vi "ABFL2dll.vi"(8 "error in (no error)":errorcluster, 11 "ABFL2 Inputs":T2) -> (0 "error out":errorcluster, 3 "ABFL2 Outputs":T1)   [LabVIEW 2016]
doc: "subroutine ABFL2dll(a, b, z, kq, ksat, ab, tbub, tdew, pbub, pdew, dlbub, dvdew, ybub, xdew, t, p, dl, dv, x,\ny, q, ierr, herr, ab_length, herr_length)\n\nGeneral flash calculation given two inputs and composition. Valid properties for the first input are temperature,\npressure, and density. Valid properties for the second are pressure, density, energy, enthalpy, entropy, or quality.\nThe character string ab specifies the inputs.\n\nThis routine accepts only two-phase states as inputs; it is intended primarily for use by the general flash routines\nsuch as THFLSH or TSFLSH. It may be called independently if the state is known to be two-phase. But beware\n- this routine does not check limits, and it will be significantly faster than TSFLSH, etc., when the bubble and\ndew point limits can be provided (ksat=1 option).\n\nThis routine calls TPFL2 within a secant-method iteration to find a solution. Initial guesses are based on the\nliquid density at the bubble point and the vapor density at the dew point.\n\nINPUTS:\n\na -- First property (either temperature, pressure, or density)\nb -- Second property (pressure, density, energy, enthalpy, entropy, or quality)\nz -- Overall composition (array of mole fractions)\nkq -- Flag specifying units for input quality when b=quality:\nksat -- Flag for bubble and dew point limits:\nab -- Character*2 string defining the inputs, e.g., 'TD' or 'PQ'\ntbub -- Bubble point temperature [K] at (P and x=z)\ntdew -- Dew point temperature [K] at (P and y=z) For temperature inputs:\npbub -- Bubble point pressure [kPa] at (T and x=z)\npdew -- Dew point pressure [kPa] at (T and y=z) For either case:\nDlbub -- Liquid density [mol/L] at bubble point\nDvdew -- Vapor density [mol/L] at dew point\nybub -- Vapor composition (array of mole fractions) at bubble point\nxdew -- Liquid composition (array of mole fractions) at dew point\nt -- Temperature [K] (if not an input)\np -- Pressure [kPa] (if not an input) \n\nOUTPUTS:\n\nt -- Temperature [K] (if not an input)\np -- Pressure [kPa] (if not an input) \n\nAll other output variables (starting with Dl) are given in the ABFLASH routine.\n\nDl -- molar density [mol/L] of the liquid phase\nDv -- molar density [mol/L] of the vapor phase \nx -- composition of liquid phase [array of mol frac]\ny -- composition of vapor phase [array of mol frac] \nq -- vapor quality on a MOLAR basis [moles vapor/total moles]\n q < 0 indicates subcooled (compressed) liquid\n q = 0 indicates saturated liquid\n q = 1 indicates saturated vapor\n q > 1 indicates superheated vapor\n q = 998 superheated vapor, but quality not defined (in most situations, t > Tc)\n q = 999 indicates supercritical state (t > Tc) and (p > Pc)\nierr -- Error flag\nherr -- Error string (character*255 variable if ierr<>0)\nab_length -- length of variable ab (default: 2)\nherr_length -- length of variable herr (default: 255)\n\nFLAGS:\n \nkq flags\n 1 Quality on molar basis (moles vapor/total moles)\n 2 Quality on mass basis (mass vapor/total mass)\nksat flags\n 1 Must provide values for the following:\n 0 Dew and bubble point limits computed here\nierr flags\n 0 Successful\n 224 Dew point calculation did not converge\n 223 Bubble point calculation did not converge\n 226 2-phase iteration did not converge"
uses:
  REFPROP.DLL
panel:
  # "REFPROP-ABFL2dll.vi"
  # "void  ABFL2dll(double *a, double *b, double *z, int32_t *kq, int32_t *ksat, CStr ab, double *tbub, double *tdew, double *pbub, double *pdew, double *Dlbub, double *Dvdew, double *ybub, double *xdew, double *t, double *p, double *Dl, double *Dv, double *x, double *y, double *q, int32_t *ierr, CStr herr, int32_t ab_length, int32_t herr_length)"
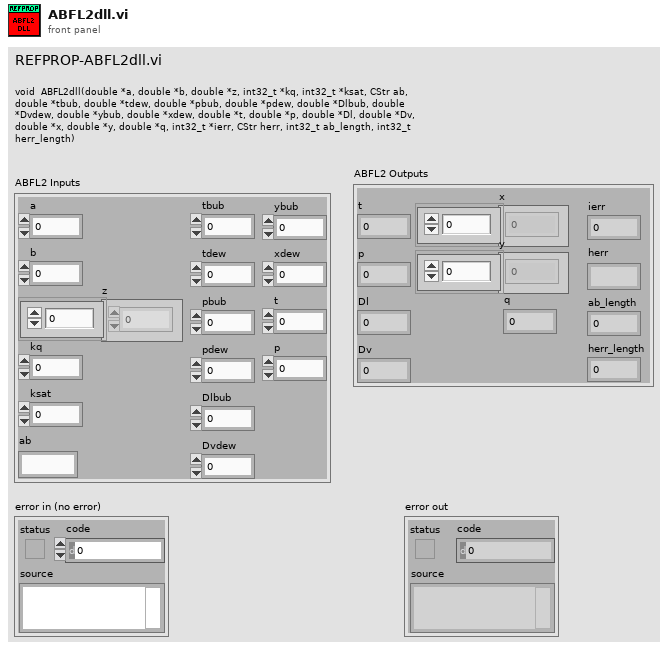
[diagram p1: front panel]
types:
  T1 = cluster{"t":dbl, "p":dbl, "Dl":dbl, "Dv":dbl, "x":dbl[], "y":dbl[], "q":dbl, "ierr":i32, "herr":string, "ab_length":i32, "herr_length":i32}
  T2 = cluster{"a":dbl, "b":dbl, "z":dbl[], "kq":i32, "ksat":i32, "ab":string, "tbub":dbl, "tdew":dbl, "pbub":dbl, "pdew":dbl, "Dlbub":dbl, "Dvdew":dbl, "ybub":dbl, "xdew":dbl, "t":dbl, "p":dbl}
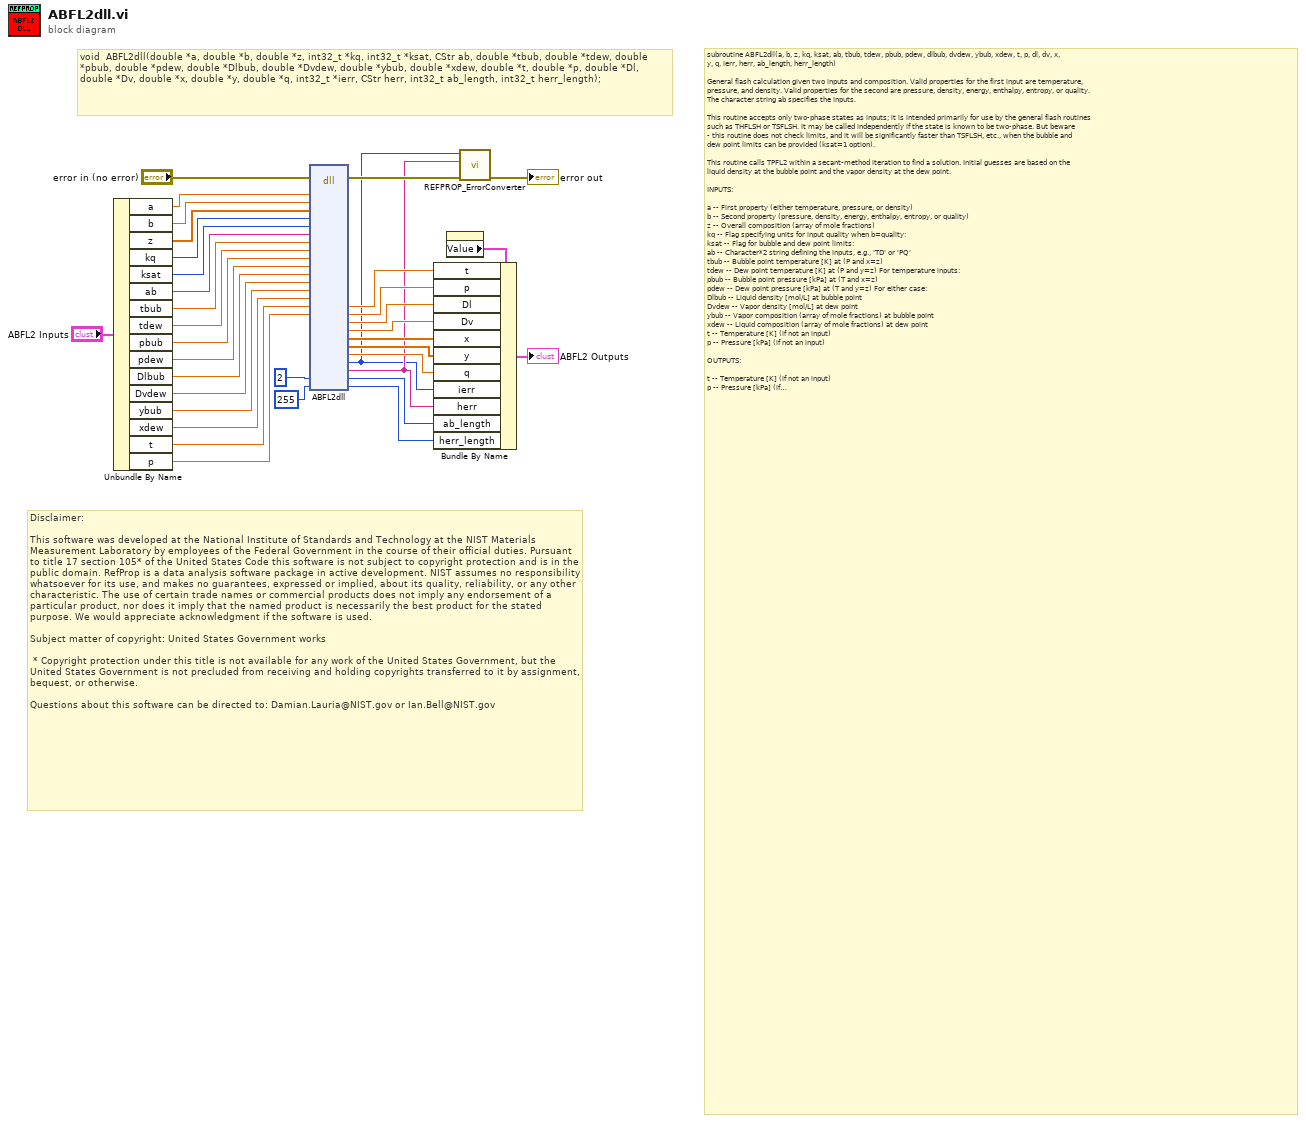
[diagram p0: block diagram]
diagram:
  # "Disclaimer:\n\nThis software was developed at the National Institute of Standards and Technology at the NIST Materials Measurement Laboratory by employees of the Federal Government in the course of their official duties. Pursuant to title 17 section 105* of the United States Code this software is not subject to copyright protection and is in the public domain. RefProp is a data analysis software package in active development. NIST assumes no responsibility whatsoever for its use, and makes no guarantees, expressed or implied, about its quality, reliability, or any other characteristic. The use of certain trade names or commercial products does not imply any endorsement of a particular product, nor does it imply that the named product is necessarily the best product for the stated purpose. We would appreciate acknowledgment if the software is used.\n \nSubject matter of copyright: United States Government works\n  \n * Copyright protection under this title is not available for any work of the United States Government, but the United States Government is not precluded from receiving and holding copyrights transferred to it by assignment, bequest, or otherwise.\n\nQuestions about this software can be directed to: Damian.Lauria@NIST.gov or Ian.Bell@NIST.gov"
  # "void  ABFL2dll(double *a, double *b, double *z, int32_t *kq, int32_t *ksat, CStr ab, double *tbub, double *tdew, double *pbub, double *pdew, double *Dlbub, double *Dvdew, double *ybub, double *xdew, double *t, double *p, double *Dl, double *Dv, double *x, double *y, double *q, int32_t *ierr, CStr herr, int32_t ab_length, int32_t herr_length);"
  # "subroutine ABFL2dll(a, b, z, kq, ksat, ab, tbub, tdew, pbub, pdew, dlbub, dvdew, ybub, xdew, t, p, dl, dv, x,\ny, q, ierr, herr, ab_length, herr_length)\n\nGeneral flash calculation given two inputs and composition. Valid properties for the first input are temperature,\npressure, and density. Valid properties for the second are pressure, density, energy, enthalpy, entropy, or quality.\nThe character string ab specifies the inputs.\n\nThis routine accepts only two-phase states as inputs; it is intended primarily for use by the general flash routines\nsuch as THFLSH or TSFLSH. It may be called independently if the state is known to be two-phase. But beware\n- this routine does not check limits, and it will be significantly faster than TSFLSH, etc., when the bubble and\ndew point limits can be provided (ksat=1 option).\n\nThis routine calls TPFL2 within a secant-method iteration to find a solution. Initial guesses are based on the\nliquid density at the bubble point and the vapor density at the dew point.\n\nINPUTS:\n\na -- First property (either temperature, pressure, or density)\nb -- Second property (pressure, density, energy, enthalpy, entropy, or quality)\nz -- Overall composition (array of mole fractions)\nkq -- Flag specifying units for input quality when b=quality:\nksat -- Flag for bubble and dew point limits:\nab -- Character*2 string defining the inputs, e.g., 'TD' or 'PQ'\ntbub -- Bubble point temperature [K] at (P and x=z)\ntdew -- Dew point temperature [K] at (P and y=z) For temperature inputs:\npbub -- Bubble point pressure [kPa] at (T and x=z)\npdew -- Dew point pressure [kPa] at (T and y=z) For either case:\nDlbub -- Liquid density [mol/L] at bubble point\nDvdew -- Vapor density [mol/L] at dew point\nybub -- Vapor composition (array of mole fractions) at bubble point\nxdew -- Liquid composition (array of mole fractions) at dew point\nt -- Temperature [K] (if not an input)\np -- Pressure [kPa] (if not an input) \n\nOUTPUTS:\n\nt -- Temperature [K] (if not an input)\np -- Pressure [kPa] (if not an input) \n\nAll other output variables (starting with Dl) are given in the ABFLASH routine.\n\nDl -- molar density [mol/L] of the liquid phase\nDv -- molar density [mol/L] of the vapor phase \nx -- composition of liquid phase [array of mol frac]\ny -- composition of vapor phase [array of mol frac] \nq -- vapor quality on a MOLAR basis [moles vapor/total moles]\n      q < 0 indicates subcooled (compressed) liquid\n      q = 0 indicates saturated liquid\n      q = 1 indicates saturated vapor\n      q > 1 indicates superheated vapor\n      q = 998 superheated vapor, but quality not defined (in most situations, t > Tc)\n      q = 999 indicates supercritical state (t > Tc) and (p > Pc)\nierr -- Error flag\nherr -- Error string (character*255 variable if ierr<>0)\nab_length -- length of variable ab (default: 2)\nherr_length -- length of variable herr (default: 255)\n\nFLAGS:\n \nkq flags\n      1 Quality on molar basis (moles vapor/total moles)\n      2 Quality on mass basis (mass vapor/total mass)\nksat flags\n      1 Must provide values for the following:\n      0 Dew and bubble point limits computed here\nierr flags\n      0 Successful\n      224 Dew point calculation did not converge\n      223 Bubble point calculation did not converge\n      226 2-phase iteration did not converge"
  n1 = Unbundle By Name("ABFL2 Inputs") -> ("a"=w20:dbl, "b"=w19:dbl, "z"=w18:dbl[], "kq"=w17:i32, "ksat"=w16:i32, "ab"=w15:string, "tbub"=w14:dbl, "tdew"=w13:dbl, "pbub"=w12:dbl, "pdew"=w11:dbl, "Dlbub"=w10:dbl, "Dvdew"=w9:dbl, "ybub"=w8:dbl, "xdew"=w7:dbl, "t"=w6:dbl, "p"=w5:dbl)
  n2 = dll-call lib="S:/009 - Testing/02 - Performance Testing/REFPROP/REFPROP.*" fn="ABFL2dll"(error in="error in (no error)", "a"=w20, "b"=w19, "z"=w18, "kq"=w17, "ksat"=w16, "ab"=w15, "tbub"=w14, "tdew"=w13, "pbub"=w12, "pdew"=w11, "Dlbub"=w10, "Dvdew"=w9, "ybub"=w8, "xdew"=w7, "t"=w6, "p"=w5, "ab_length"=2, "herr_length"=255) -> (error out=w35:errorcluster, "t"=w29:dbl, "p"=w28:dbl, "Dl"=w27:dbl, "Dv"=w26:dbl, "x"=w25:dbl[], "y"=w24:dbl[], "q"=w23:dbl, "ierr"=w1:i32, "herr"=w2:string, "ab_length"=w22:i32, "herr_length"=w21:i32)  [unwired: 24 in, 1 out]
  n3 = property on="ABFL2 Outputs" class="Clust (strict)"() -> ("Value"=w4:T1)  [unwired: 2 in, 2 out]
  n4 = Bundle By Name(cluster=w4, "t"=w29, "p"=w28, "Dl"=w27, "Dv"=w26, "x"=w25, "y"=w24, "q"=w23, "ierr"=w1, "herr"=w2, "ab_length"=w22, "herr_length"=w21) -> (→"ABFL2 Outputs":T1)
  n5 = call "REFPROP_ErrorConverter.vi"("error in (no error)"=w35, "Error Message"=w2, "Error Code"=w1) -> ("error out"=→"error out":errorcluster)  [unwired: 8 in]
